vi "LC_BESS_React_Ctrl.vi"   [LabVIEW 2016]
uses:
  LabVIEW Data/MathScriptVIs/MCStatic_36913153632_137dbbc8b62ff179ad17ce13afb809c8.vi
  <instcachedir>/0/MCStatic_36913153632_137dbbc8b62ff179ad17ce13afb809c8_7337D6D141B744C0ACEB8CFFCA4DAD86.lvgen/MCStatic_36913153632_137dbbc8b62ff179ad17ce13afb809c8_7337D6D141B744C0ACEB8CFFCA4DAD86_001.vi
  <vilib>/imath/engines/lvmath2/RunTimeEngine/NodeEndStatement/NIMS_NodeEndStatement_Output.vi
  <instcachedir>/0/NIMS_NodeEndStatement_Output_53EC0D466D134D7ABD903AC30B43404B.lvgen/NIMS_NodeEndStatement_Output_53EC0D466D134D7ABD903AC30B43404B_001.vi
  <vilib>/imath/engines/lvmath2/RunTimeEngine/ErrorHandling/NIMS_Finalize Error.vi
  PIcontroller.m
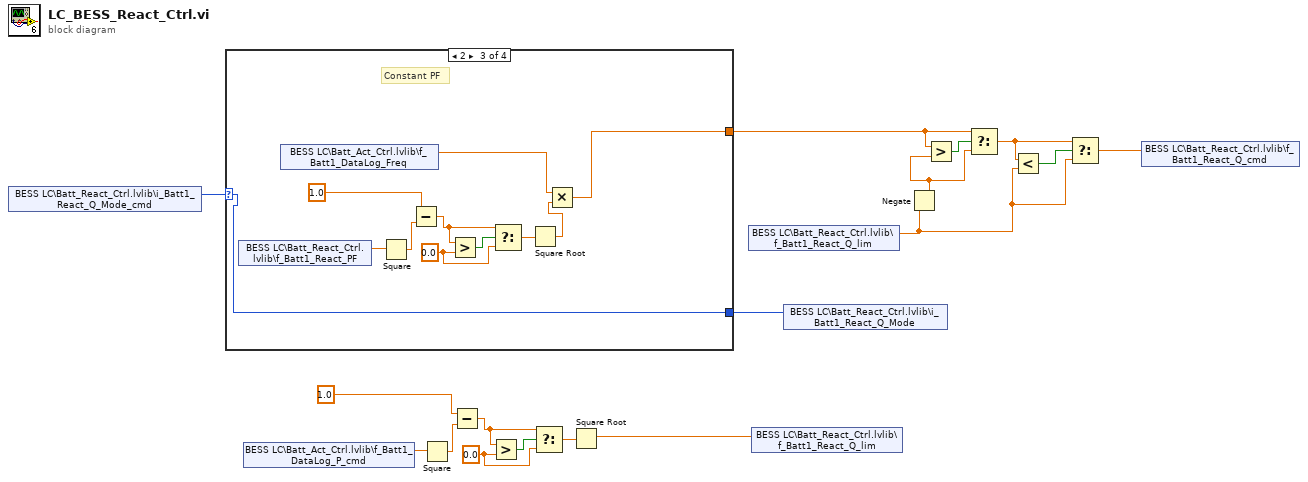
[diagram p0: block diagram]
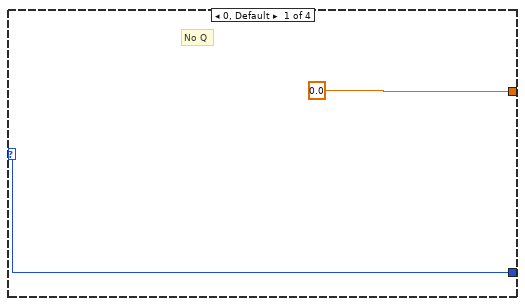
[diagram p2: hidden frame]
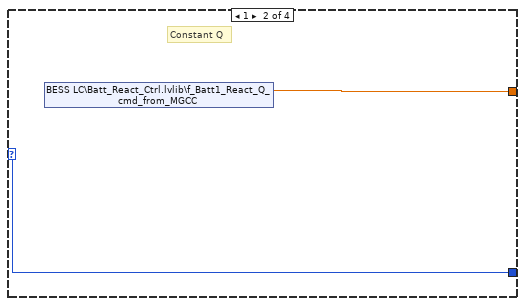
[diagram p3: hidden frame]
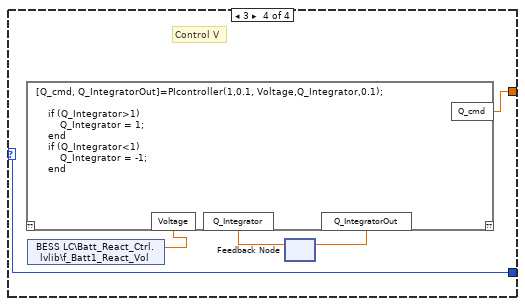
[diagram p4: hidden frame]
diagram:
  w1 = 0.0 ("y")
  n1 = shared-variable "BESS LC\\Batt_React_Ctrl.lvlib\\i_Batt1_React_Q_Mode_cmd"() -> (w17:i16)  [unwired: 1 in, 1 out]
  n2 = case shown="2" w17 {
    selector: w17 -> [w18 w20 w22 w37]
    tunnel: [0.0 ("f_Batt1_React_Q_cmd") w21 w23 w36] -> w14
    tunnel: [w18 w20 w22 w37] -> w16
    frame 0, Default {
      # "No Q"
    }
    frame 1 {
      # "Constant Q"
      n3 = shared-variable "BESS LC\\Batt_React_Ctrl.lvlib\\f_Batt1_React_Q_cmd_from_MGCC"() -> (w21:dbl)  [unwired: 1 in, 1 out]
    }
    frame 2 {
      w26 = 0.0 ("y")
      # "Constant PF"
      n4 = shared-variable "BESS LC\\Batt_React_Ctrl.lvlib\\f_Batt1_React_PF"() -> (w32:dbl)  [unwired: 1 in, 1 out]
      n5 = shared-variable "BESS LC\\Batt_Act_Ctrl.lvlib\\f_Batt1_DataLog_Freq"() -> (w25:dbl)  [unwired: 1 in, 1 out]
      n6 = Square(x=w32) -> (x^2=w31:dbl)
      n7 = Subtract(x=1.0 ("f_Batt1_React_Q_lim"), y=w31) -> (x-y=w27:dbl)
      n8 = Greater?(x=w27, y=w26) -> (0:w29:bool)
      n9 = Select(t=w27, s=w29, f=w26) -> (s? t:f=w28:dbl)
      n10 = Square Root(x=w28) -> (sqrt(x)=w24:dbl)
      n11 = Multiply(x=w25, y=w24) -> (x*y=w23:dbl)
    }
    frame 3 {
      # "Control V"
      n12 = shared-variable "BESS LC\\Batt_React_Ctrl.lvlib\\f_Batt1_React_Vol"() -> (w33:dbl)  [unwired: 1 in, 1 out]
      n13 = feedback #1() -> (w34:dbl)  [unwired: 1 in]
      n14 = mathscript code="[Q_cmd, Q_IntegratorOut]=PIcontroller(1,0.1, Voltage,Q_Integrator,0.1);\n   \n    if (Q_Integrator>1)\n        Q_Integrator = 1;\n    end \n    if (Q_Integrator<1)\n        Q_Integrator = -1;\n    end"("Voltage"=w33, "Q_Integrator"=w34) -> ("Q_cmd"=w36:dbl, "Q_IntegratorOut"=w35:dbl)  [unwired: 1 in, 1 out]
      n15 = feedback-in #1(w35) -> ()
    }
  }
  n16 = shared-variable "BESS LC\\Batt_Act_Ctrl.lvlib\\f_Batt1_DataLog_P_cmd"() -> (w8:dbl)  [unwired: 1 in, 1 out]
  n17 = Square(x=w8) -> (x^2=w7:dbl)
  n18 = Subtract(x=1.0 ("f_Batt1_React_Q_lim"), y=w7) -> (x-y=w2:dbl)
  n19 = Greater?(x=w2, y=w1) -> (0:w4:bool)
  n20 = Select(t=w2, s=w4, f=w1) -> (s? t:f=w3:dbl)
  n21 = Square Root(x=w3) -> (sqrt(x)=w5:dbl)
  n22 = shared-variable "BESS LC\\Batt_React_Ctrl.lvlib\\f_Batt1_React_Q_lim"() -> (w11:dbl)  [unwired: 1 in, 1 out]
  n23 = shared-variable "BESS LC\\Batt_React_Ctrl.lvlib\\f_Batt1_React_Q_lim"(w5) -> ()  [unwired: 1 in, 1 out]
  n24 = shared-variable "BESS LC\\Batt_React_Ctrl.lvlib\\i_Batt1_React_Q_Mode"(w16) -> ()  [unwired: 1 in, 1 out]
  n25 = Negate(x=w11) -> (-x=w13:dbl)
  n26 = Greater?(x=w14, y=w13) -> (0:w15:bool)
  n27 = Select(t=w14, s=w15, f=w13) -> (s? t:f=w12:dbl)
  n28 = Less?(x=w12, y=w11) -> (x < y?=w10:bool)
  n29 = Select(t=w12, s=w10, f=w11) -> (s? t:f=w9:dbl)
  n30 = shared-variable "BESS LC\\Batt_React_Ctrl.lvlib\\f_Batt1_React_Q_cmd"(w9) -> ()  [unwired: 1 in, 1 out]
